vi "Global Write.vi"(8 "error in (no error)":errorcluster, 10 "Incoming Cluster":T1, 11 "Pump Number In":i32) -> (0 "error out":errorcluster, 3 "Pump Number Out":i32)   [LabVIEW 2018, in "Ismatec 4308.lvlib"]
uses:
  Ismatec 4308.lvlib
  Ismatec 4083 Global Element.ctl
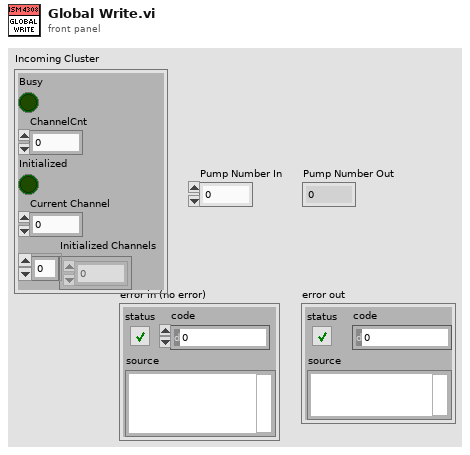
[diagram p1: front panel]
types:
  T1 = typedef "Ismatec 4308.lvlib/Ismatec 4083 Global Element.ctl" = cluster{"Busy":bool, "ChannelCnt":dbl, "Initialized":bool, "Current Channel":dbl, "Initialized Channels":dbl[]}
  T2 = cluster{"Busy":bool, "ChannelCnt":dbl, "Initialized":bool, "Current Channel":dbl, "Initialized Channels":dbl[]}[]
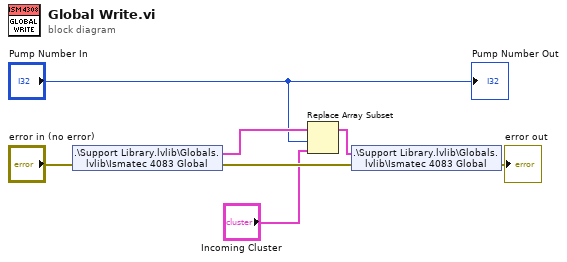
[diagram p0: block diagram]
diagram:
  n1 = shared-variable ".\\Support Library.lvlib\\Globals.lvlib\\Ismatec 4083 Global"(error in="error in (no error)") -> (w3:T2, error out=w7:errorcluster)
  n2 = Replace Array Subset(array=w3, new element="Incoming Cluster", index="Pump Number In") -> (w4:T2)
  n3 = shared-variable ".\\Support Library.lvlib\\Globals.lvlib\\Ismatec 4083 Global"(w4, error in=w7) -> (error out=→"error out":errorcluster)
  "Pump Number Out" <- "Pump Number In"
